vi "FGEN Edit.vi"(8 "error in":errorcluster, 10 "Sequence Context In":refnum<k7>, 11 "FGENIn":T1={"Enable Output"=FALSE, "Amplitude (Vp-p) "=1.0, "Frequency (Hz)"=1000000.0, "DC Offset (V)"=0.0, "Start Phase"=0.0, "Standard Waveform"=0, "FGEN Operation"=enum."Configure", "Active Channel"=""} {"Standard Waveform" scale=0.0..6.0; "DC Offset (V)" min=-6.0 max=6.0 scale=-6.0..6.0 scale format="%_1p"; "Frequency (Hz)" min=9000.0 max=100000000.0 scale=0.0..100000000.0 scale format="%_1p"; "Amplitude (Vp-p)" min=0.0 max=12.0 scale=0.0..12.0 scale format="%.1f"}) -> (0 "error out":errorcluster, 2 "Report Text":string, 3 "FGENOut":T1={"Enable Output"=FALSE, "Amplitude (Vp-p) "=1.0, "Frequency (Hz)"=1000000.0, "DC Offset (V)"=0.0, "Start Phase"=0.0, "Standard Waveform"=0, "FGEN Operation"=enum."Configure", "Active Channel"=""} {"Standard Waveform" scale=0.0..6.0; "DC Offset (V)" min=-6.0 max=6.0 scale=-6.0..6.0 scale format="%_1p"; "Frequency (Hz)" min=9000.0 max=100000000.0 scale=0.0..100000000.0 scale format="%_1p"; "Amplitude (Vp-p)" min=0.0 max=12.0 scale=0.0..12.0 scale format="%.1f"})   [LabVIEW 2023, in "LTT_TeststandSteptypes.lvlib"]
uses:
  LTT_TeststandSteptypes.lvlib
  Control/FGEN Data.ctl
  <vilib>/addons/TestStand/_TSUtility.llb/TestStand - Start Modal Dialog (Sequence Context).vi
  <vilib>/addons/TestStand/_TSUtility.llb/TestStand - End Modal Dialog (Sequence Context).vi
panel:
  in  "FGEN Operation":T2(tab)
  in  "Channel Number":string(combo)
  in  "Standard Waveform":u16(slide) scale=0.0..6.0
  in  "Start Phase":dbl
  in  "DC Offset (V)":dbl(knob) min=-6.0 max=6.0 scale=-6.0..6.0 scale format="%_1p"
  in  "Frequency (Hz)":dbl(knob)=1000000.0 min=9000.0 max=100000000.0 scale=0.0..100000000.0 scale format="%_1p"
  in  "Amplitude (Vp-p)":dbl(knob)=1.0 min=0.0 max=12.0 scale=0.0..12.0 scale format="%.1f"
  in  "Enable Output":bool
  in  "Close":bool
  in  "OK":bool
  # "Init for Function Generator Configuration read from database"
  # "Self Test is Enabled by selecting this opeartion"
  # "Start for Function Generator"
  # "Stop for Function Generator"
  # "Measure the  Actual Frequency and Actual Amplitude, Actual DC Offset, Actual Standard Waveform."
  # "FGEN Close Operation will be executing by selecting this opeartion"
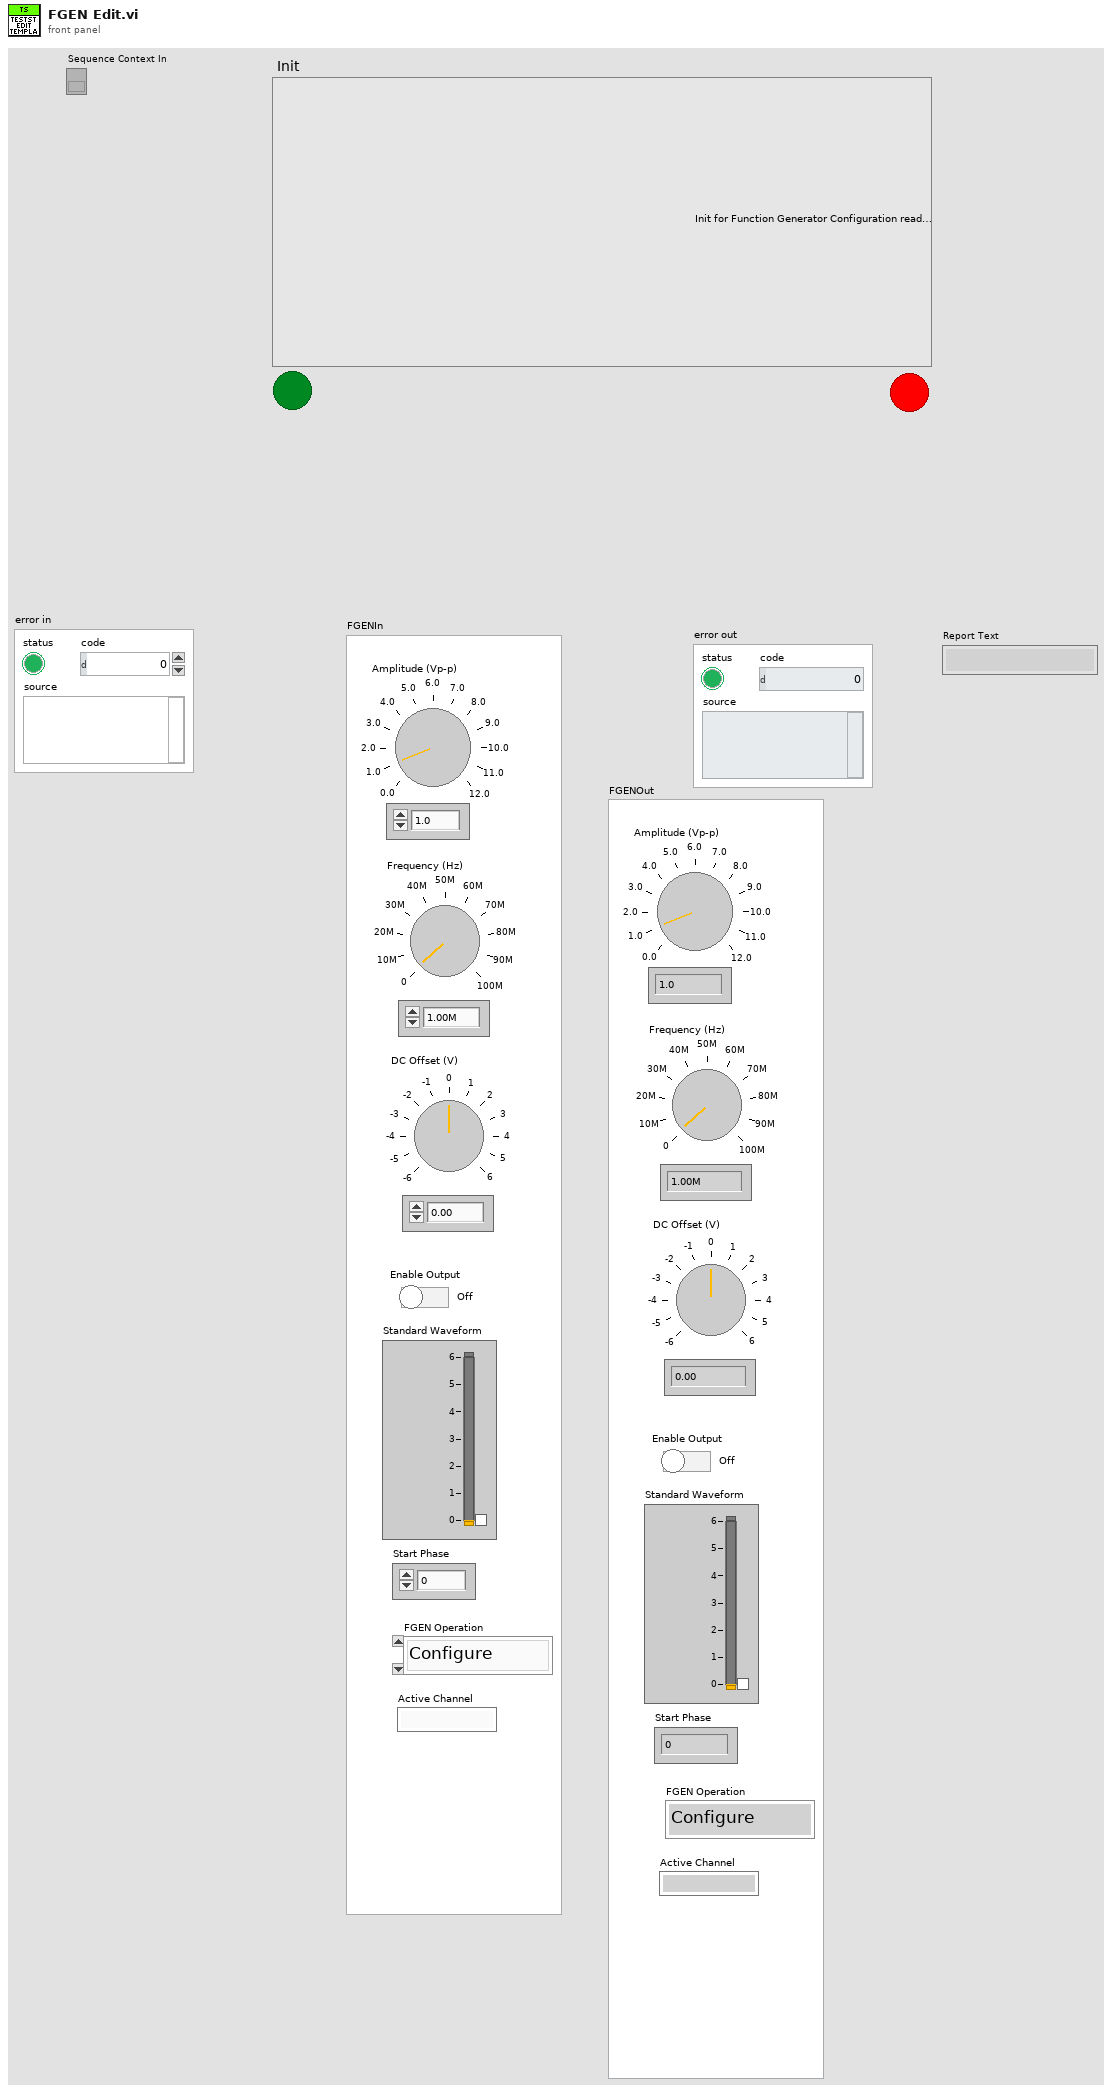
[diagram p1: front panel]
types:
  T1 = typedef "LTT_TeststandSteptypes.lvlib/FGEN Data.ctl" = cluster{"Enable Output":bool, "Amplitude (Vp-p) ":dbl, "Frequency (Hz)":dbl, "DC Offset (V)":dbl, "Start Phase":dbl, "Standard Waveform":u16, "FGEN Operation":enum32{"Init", "Self Test", "Configure Channel", "Configure", "Start", "Stop", "Measure", "Close"}, "Active Channel":string}
  T2 = enum32{"Init", "Self Test", "Configure Channel", "Configure", "Start", "Stop", "Measure", "Close"}
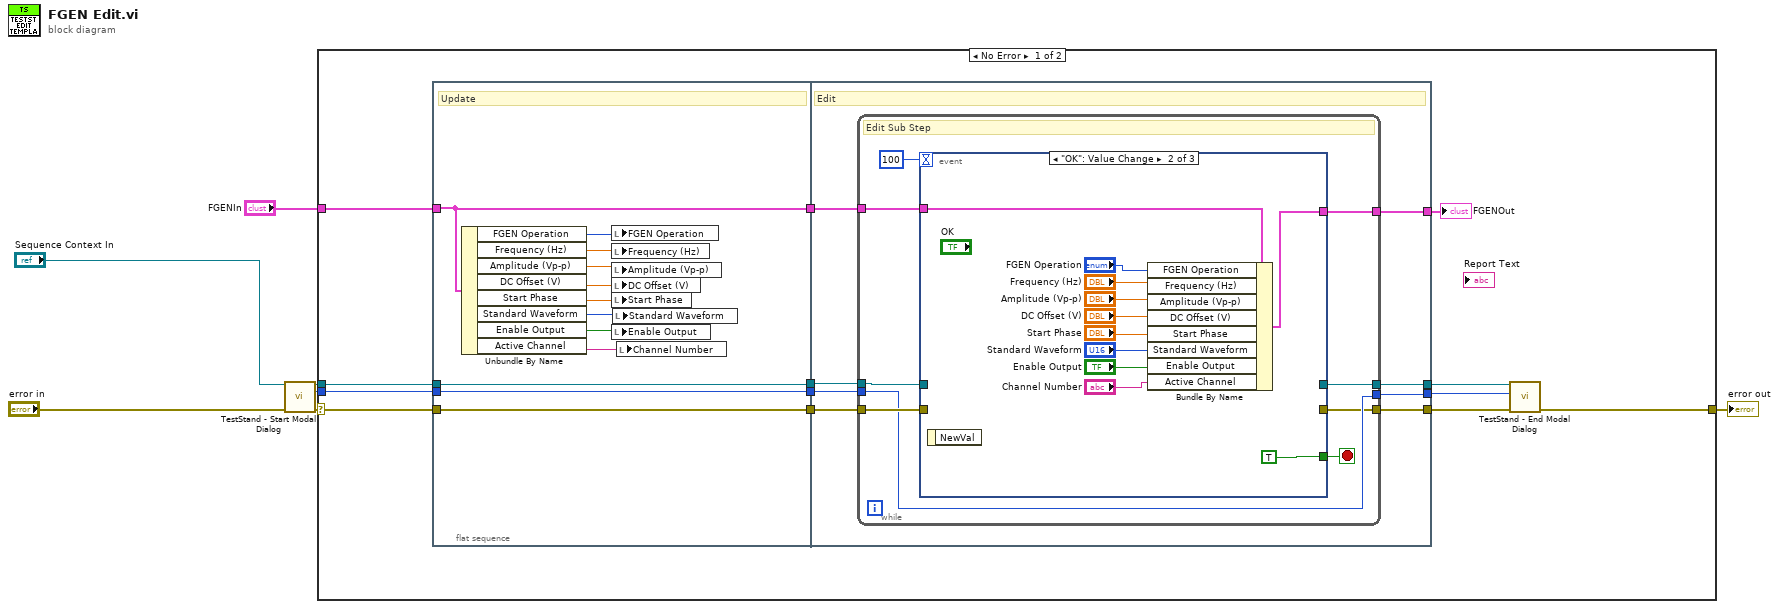
[diagram p0: block diagram]
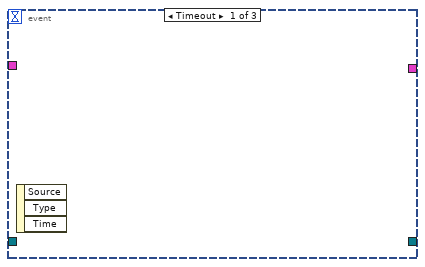
[diagram p2: hidden frame]
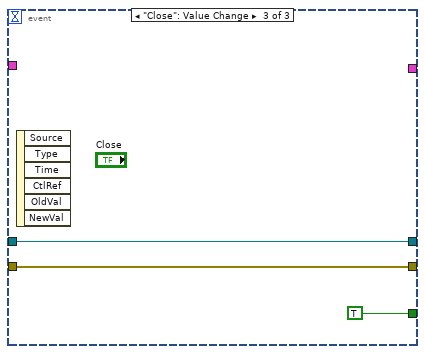
[diagram p3: hidden frame]
diagram:
  n1 = call-poly <vilib>:"TestStand - Start Modal Dialog.vi"("Sequence Context In"="Sequence Context In", "error in (no error)"="error in") -> ("Sequence Context Out"=w4:refnum<k7>, "Modal ID"=w3:i32, "error out"=w5:errorcluster)  [unwired: 9 in, 2 out]
  n2 = case shown="No Error" w5 {
    selector: w5 -> [w17 w64]
    tunnel: w4 -> [w14 _]
    tunnel: w3 -> [w13 _]
    tunnel: [w15 w64] -> w2
    tunnel: "FGENIn" -> [w9 _]
    frame No Error {
      n3 = flat-sequence {
        tunnel: w17 -> [w32]
        tunnel: [w32] -> w20
        tunnel: w14 -> [w31]
        tunnel: w13 -> [w30]
        tunnel: [w31] -> w19
        tunnel: [w30] -> w18
        tunnel: [w29] -> w10
        tunnel: w9 -> [w29]
        tunnel: w20 -> [w38]
        tunnel: [w36] -> w16
        tunnel: w19 -> [w40]
        tunnel: w18 -> [w39]
        tunnel: [w37] -> w12
        tunnel: [w35] -> w11
        tunnel: w10 -> [w34]
        tunnel: [w33] -> w8
        frame #0 {
          # "Update"
          n4 = Unbundle By Name(w29) -> ("FGEN Operation"=w28:T2, "Frequency (Hz)"=w27:dbl, "Amplitude (Vp-p)"=w26:dbl, "DC Offset (V)"=w25:dbl, "Start Phase"=w24:dbl, "Standard Waveform"=w23:u16, "Enable Output"=w22:bool, "Active Channel"=w21:string)
          n5 = local write "FGEN Operation"(w28) -> ()
          n6 = local write "Frequency (Hz)"(w27) -> ()
          n7 = local write "Amplitude (Vp-p)"(w26) -> ()
          n8 = local write "DC Offset (V)"(w25) -> ()
          n9 = local write "Start Phase"(w24) -> ()
          n10 = local write "Enable Output"(w22) -> ()
          n11 = local write "Standard Waveform"(w23) -> ()
          n12 = local write "Channel Number"(w21) -> ()
        }
        frame #1 {
          # "Edit"
          n13 = while {
            tunnel: w40 -> [w47]
            tunnel: w39 -> [w44]
            tunnel: w38 -> [w45]
            tunnel: [w46] -> w35
            tunnel: [w44] -> w37
            tunnel: [w43] -> w36
            tunnel: w34 -> [w42]
            tunnel: [w41] -> w33
            stop <- w48 stop-if-true
            # "Edit Sub Step"
            n14 = event shown="[1] \"OK\": Value Change" {
              selector: _ -> [_ _ _]
              dyn-events: _ -> [_ _ _]
              timeout: 100 -> [_ _ _]
              tunnel: [_ TRUE TRUE] -> w48
              tunnel: [_ _ w62] -> w46
              tunnel: w47 -> [_ _ w62]
              tunnel: w45 -> [_ _ w61]
              tunnel: [_ _ w61] -> w43
              tunnel: w42 -> [_ w59 _]
              tunnel: [_ w58 _] -> w41
              event Timeout {
                n15 = event-data() -> ()  [unwired: 1 in, 3 out]
              }
              event "OK": Value Change {
                n16 = event-data() -> ()  [unwired: 1 in, 1 out]
                n17 = Bundle By Name(cluster=w59, "FGEN Operation"="FGEN Operation", "Frequency (Hz)"="Frequency (Hz)", "Amplitude (Vp-p)"="Amplitude (Vp-p)", "DC Offset (V)"="DC Offset (V)", "Start Phase"="Start Phase", "Standard Waveform"="Standard Waveform", "Enable Output"="Enable Output", "Active Channel"="Channel Number") -> (w58:T1)
              }
              event "Close": Value Change {
                n18 = event-data() -> ()  [unwired: 1 in, 6 out]
              }
            }
          }
        }
      }
      n19 = call-poly <vilib>:"TestStand - End Modal Dialog.vi"("Sequence Context In"=w11, "Modal ID"=w12, "error in (no error)"=w16) -> ("error out"=w15:errorcluster)  [unwired: 12 in]
      "FGENOut" <- w8
    }
    frame Error {
    }
  }
  "error out" <- w2
